vi "PV Digiline Display settings.vi"(7 "Adress of unit":u16=1 max=999 step=1, 8 "error in (no error)":errorcluster, 9 "Parameter\nread only<->describe":bool, 10 "Display settings":u16(ring)=4 items=[" Display 0°"=4, " Display 180°"=6, " Pressure [hPa]"=8, " 0° [hPa]"=12, " 180 ° [hPa]"=14, " Pressure [mbar]"=16, " 0° [mbar]"=20, " 180° [mbar]"=22, " Pressure [Torr]"=24, " 0° [Torr]"=28, " 180° [Torr]"=30], 11 "VISA session":refnum<visa-resource-name>) -> (0 "error out":errorcluster, 2 "response (data)":string, 3 "dup VISA session":refnum<visa-resource-name>)   [LabVIEW 2021, in "Pfeiffer Vacuum.lvlib"]
doc: "There are 1 parameter available at a time. VI only for DigiLine gauges with display.\n\n0 - Display settings (default)\n\nNote: The 1 control right of this one will set the appropriate values for the selected parameter. Any settings for an parameter that is not selected will be ignored. If a value is out of range, it will be changed to either the upper or the lower limit of the range."
uses:
  <instrlib>/Pfeiffer Vacuum/Pfeiffer Vacuum.lvlib
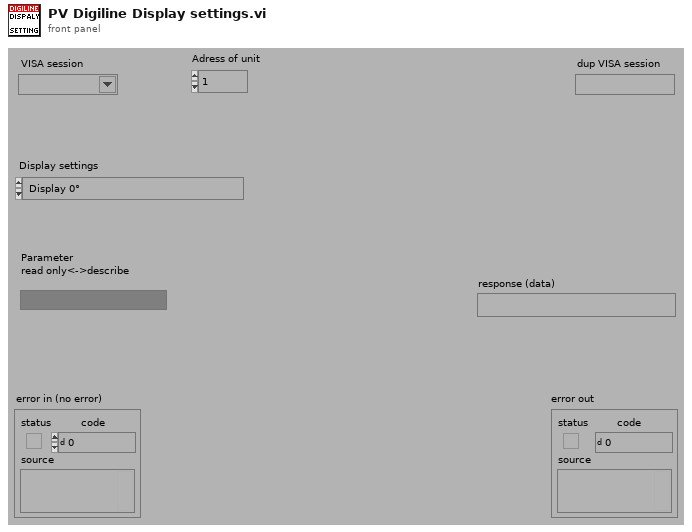
[diagram p1: front panel]
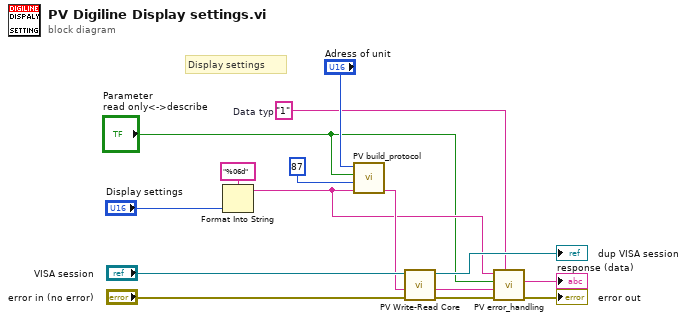
[diagram p0: block diagram]
diagram:
  w6 = "1"  # Data typ
  # "Display settings"
  n1 = Format Into String(format string="%06d" ("Format-String"), "Display settings") -> (resulting string=w3:string)  [unwired: 2 in, 1 out]
  n2 = call <instrlib>:"PV build_protocol.vi"("Data"=w3, "Parameter-number"=u16 87, "parameter\nread<->describe"="Parameter\nread only<->describe", "Adress"="Adress of unit") -> ("output"=w10:string)  [unwired: 3 in]
  n3 = call <instrlib>:"PV Write-Read Core.vi"("error in"="error in (no error)", "Write data in"=w10, "VISA session"="VISA session") -> ("error out"=w7:errorcluster, "response (data) out"=w8:string, "dup VISA session"=→"dup VISA session":refnum<visa-resource-name>)  [unwired: 2 in]
  n4 = call <instrlib>:"PV error_handling.vi"("Data Typ in"=w6, "error in"=w7, "response (data) in"=w8, "Parameter\nread only<->describe"="Parameter\nread only<->describe", "data in"=w3) -> ("error out"=→"error out":errorcluster, "Data out"=→"response (data)":string)  [unwired: 4 in, 1 out]
